vi "ArcadeScaleCurve.vi"(10 "Direction":dbl format="%#_13g") -> (2 "Scale":dbl)   [LabVIEW 2015]
doc: "Determines the scale based on the given direction by using this formula: scale = cos(pi*abs(direction)). Therefore, the range is [-1, 1]."
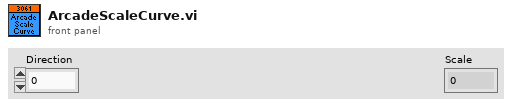
[diagram p1: front panel]
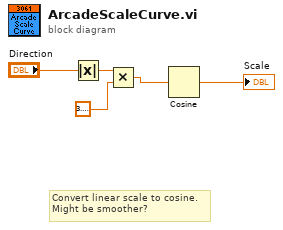
[diagram p0: block diagram]
diagram:
  # "Convert linear scale to cosine.\nMight be smoother?"
  n1 = Absolute Value(x="Direction") -> (abs(x)=w2:dbl)
  n2 = Multiply(x=w2, y=3.141592653589793) -> (x*y=w4:dbl)
  n3 = Cosine(x=w4) -> (cos(x)=→"Scale":dbl)
